vi "configure channel.vi"(7 "EthernetIP configuration":refnum<class "EIP Tags Configuration.lvclass">, 8 "error in":errorcluster, 10 "line item in":T2, 11 "engine configuration in":refnum<class "engine configuration.lvclass">) -> (0 "error out":errorcluster, 1 "success":bool, 2 "line item out":T2, 5 "changed":bool)   [LabVIEW 2013, in "EIP Tags editor node.lvclass"]
uses:
  EIP Tags editor node.lvclass
  table line.ctl
  channel/EIP Tags Channel.lvclass
  <vilib>/NI/Module Execution Interface/Engine Configuration/engine configuration.lvclass
  configuration/EIP Tags Configuration.lvclass
  tag direction.ctl
  configuration/EIP Tags Configuration.lvclass/EIP Tags Configuration.ctl
  <vilib>/NI/Configuration Framework/serializable configuration/NISE_CEF_serializable configuration.lvclass/NISE_CEF_serializable configuration.ctl
  <vilib>/NI/Tag Bus Module Framework/channel/channel classification.ctl
  <vilib>/NI/Tag Bus Module Framework/channel/TBM channel.lvclass/TBM channel.ctl
  <vilib>/NI/Tag Bus/tag/tag descriptor.lvclass/tag descriptor.ctl
  channel/EIP Tags Channel.lvclass/EIP Tags Channel.ctl
  <vilib>/NI/Tag Bus/tag/Data Type.ctl
  configuration/Read EIP tags.vi
  <vilib>/NI/Configuration Framework/serializable configuration/Read UID.vi
  <vilib>/NI/Tag Bus Module Framework/channel/Read channel classification.vi
  <vilib>/NI/Tag Bus/tag/read tag name.vi
  channel/Read element.vi
  channel/Read EIP Tag UUID.vi
  <vilib>/NI/Tag Bus/tag/write tag name.vi
  <vilib>/NI/Tag Bus Module Framework/channel/Write channel classification.vi
  channel/Write EIP Tag UUID.vi
  <vilib>/NI/Tag Bus/tag/read data type.vi
  <vilib>/NI/Tag Bus/tag/write data type.vi
  channel/Write element.vi
  <vilib>/Utility/LVClass/Get LV Class Name.vi
  <vilib>/NI/Configuration Framework/error generator.vi
  <vilib>/NI/Tag Bus Module Framework/channel/TBM channel.lvclass
  <vilib>/NI/Tag Bus/tag/tag descriptor.lvclass
panel:
  in  "Store full array":bool
  in  "direction":T1
  in  "refresh tags":bool
  in  "TBDF Tag":i32(listbox)
  in  "EIP Tag":i32(listbox)
  out "problem":string
  in  "Element Index":i32
  in  "Channel Name":string
  in  "cancel":bool
  in  "ok":bool
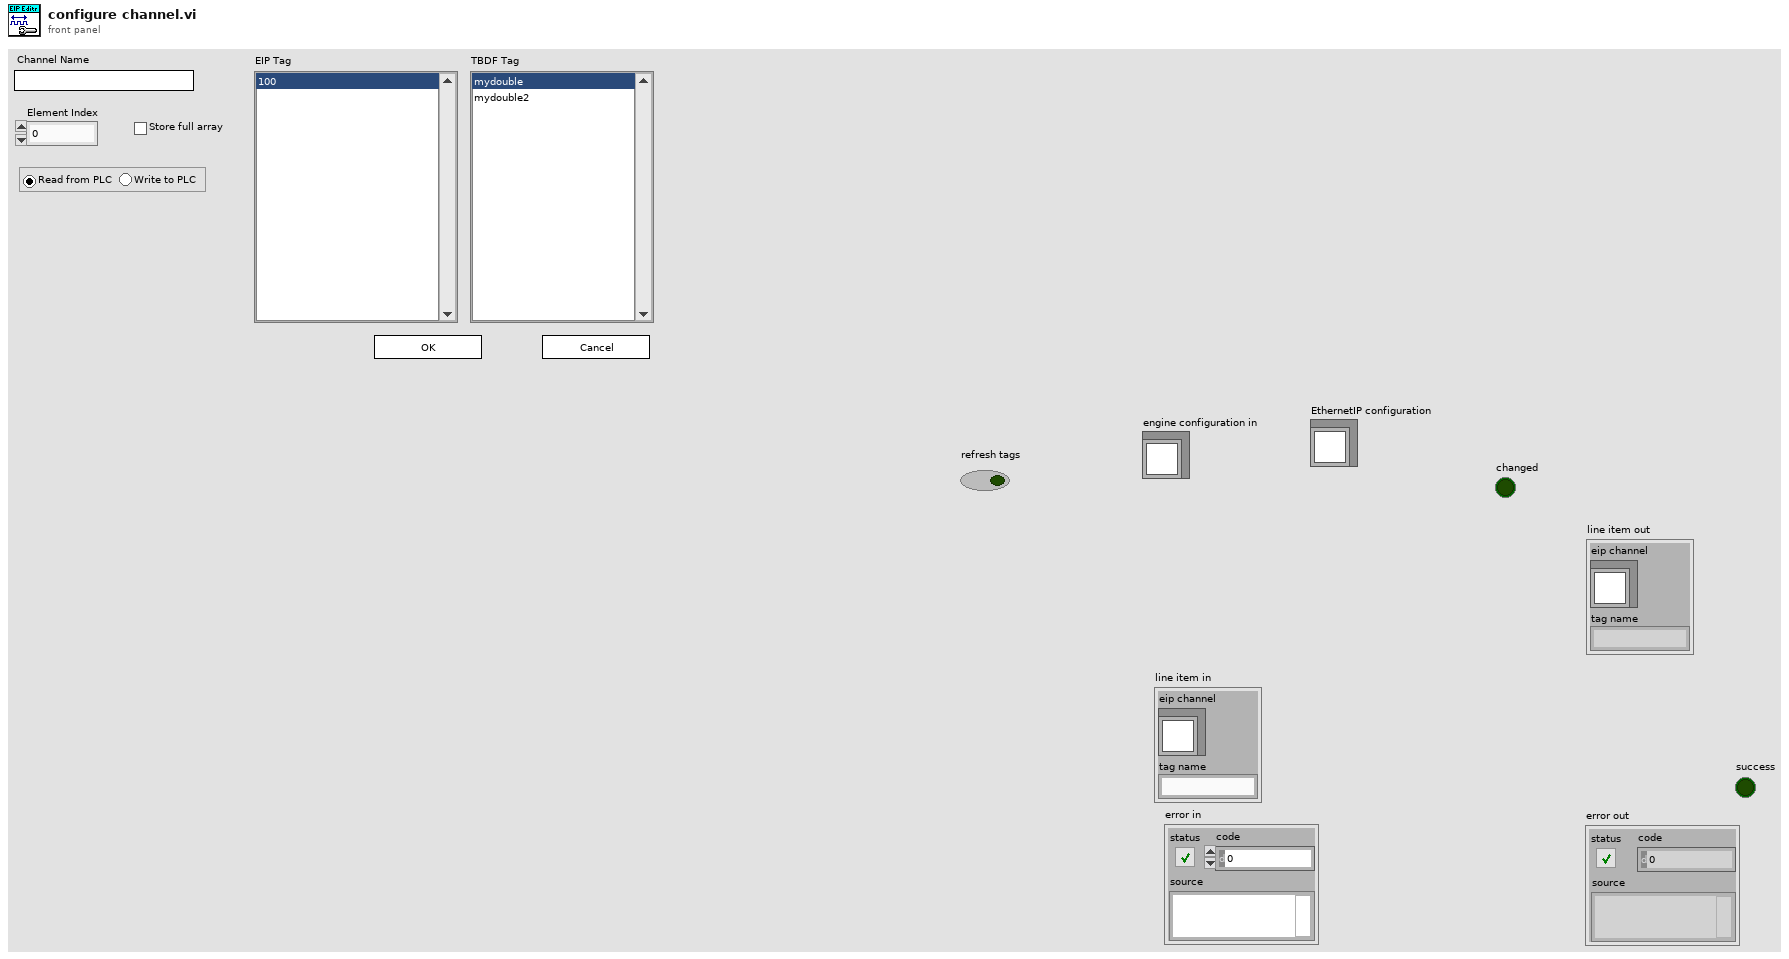
[diagram p1: front panel]
types:
  T1 = typedef "EIP Tags editor node.lvclass/tag direction.ctl" = enum32{"Read from PLC", "Write to PLC"}
  T2 = typedef "EIP Tags editor node.lvclass/table line.ctl" = cluster{"eip channel":refnum<class "EIP Tags Channel.lvclass">, "tag name":string}
  T3 = enum32{"Invalid", "Standard", "Closed", "Hidden", "Minimized", "Maximized"}
  T4 = enum32{"Invalid", "Default", "Floating", "Floating/Auto-Hide", "Modal"}
  T5 = typedef "TBM channel.lvclass/channel classification.ctl" = enum16{"input data", "output data", "processing parameter", "processing result"}
  T6 = enum8{"Enabled", "Disabled", "Disabled and Grayed Out"}
  T7 = typedef "tag bus.lvlib/tag descriptor.lvclass/Data Type.ctl" = enum16{"Double", "Single", "I64", "I32", "I16", "I8", "U64", "U32", "U16", "U8", "Boolean", "String", "Array of Double", "Array of Single", "Array of I64", "Array of I32", "Array of I16", "Array of I8", "Array of U64", "Array of U32", "Array of U16", "Array of U8", "Array of Boolean", "Array of String"}
  T8 = typedef "EIP Tags Configuration.lvclass/eip tag definition.ctl" = cluster{"eip tag types":T9, "unique tag name":string, "Number of Elements":u32}
  T9 = typedef "EIP Tags Configuration.lvclass/eip tag types.ctl" = enum16{"SINT", "INT", "DINT", "REAL", "BOOL", "STRING"}
  T10 = cluster{"unique tag name":string, "tag spec":T8}[]
  T11 = enum32{"invalid app kind", "Development System", "Run Time System", "Student Edition", "Embedded LabVIEW", "Evaluation", "Custom"}
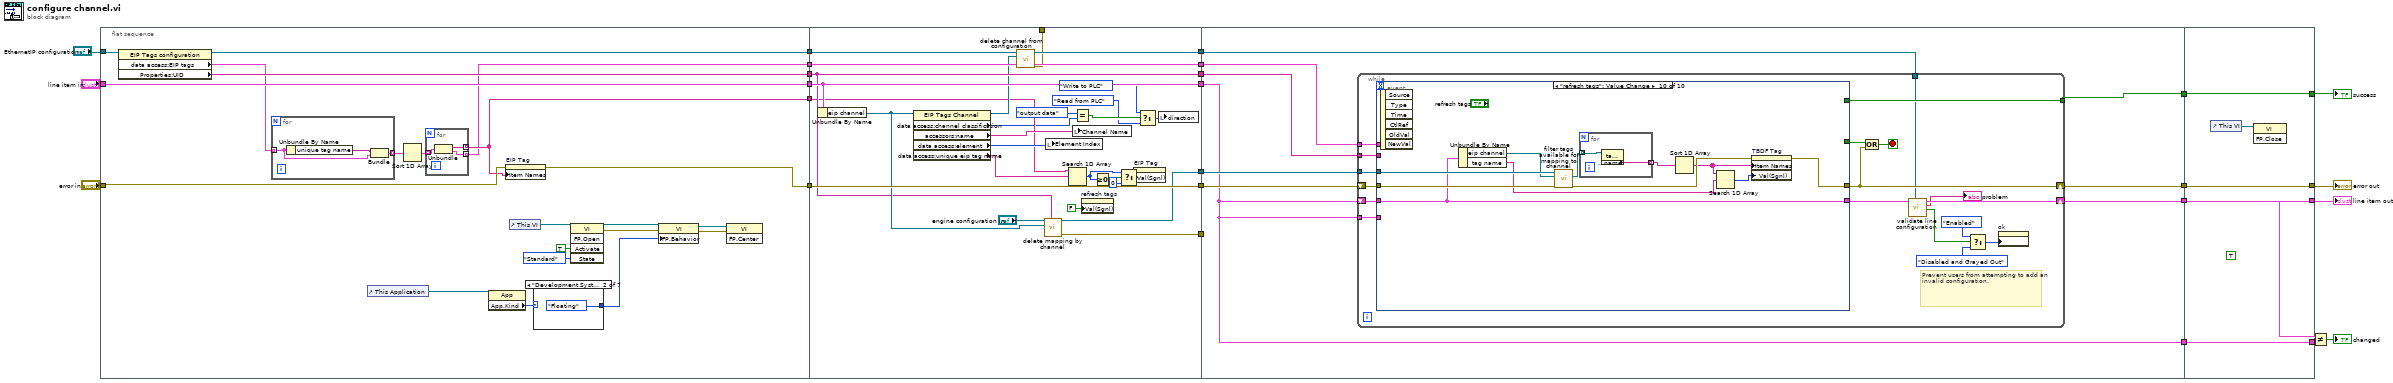
[diagram p0: block diagram]
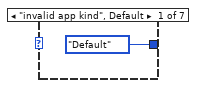
[diagram p2: hidden frame]
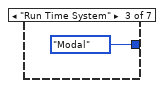
[diagram p3: hidden frame]
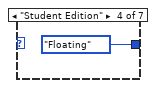
[diagram p4: hidden frame]
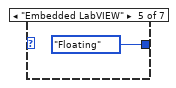
[diagram p5: hidden frame]
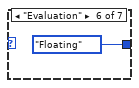
[diagram p6: hidden frame]
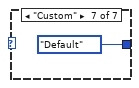
[diagram p7: hidden frame]
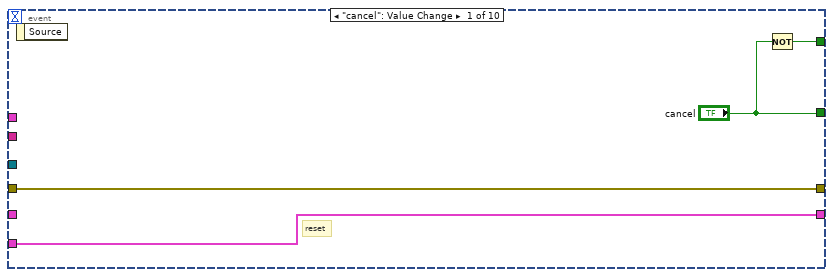
[diagram p8: hidden frame]
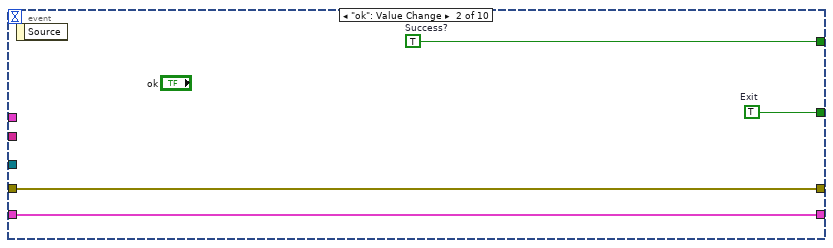
[diagram p9: hidden frame]
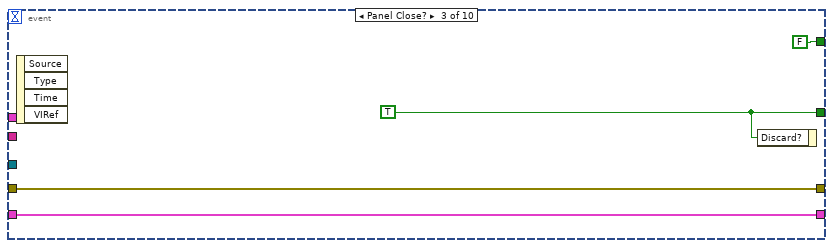
[diagram p10: hidden frame]
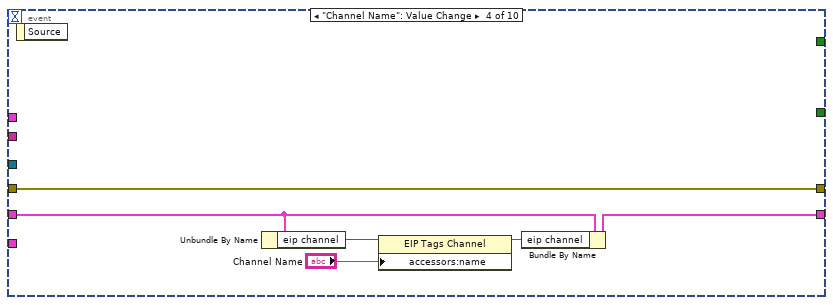
[diagram p11: hidden frame]
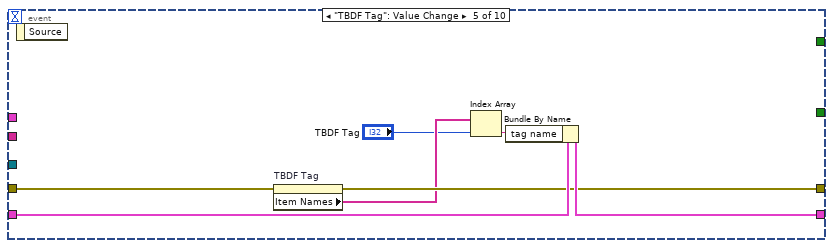
[diagram p12: hidden frame]
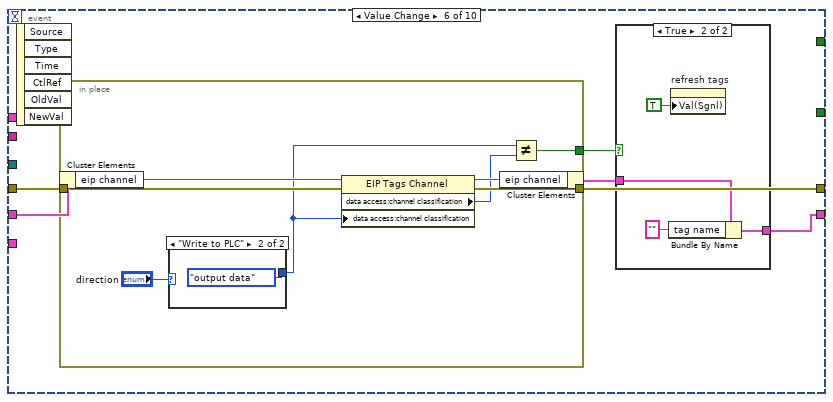
[diagram p13: hidden frame]
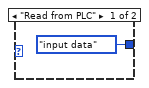
[diagram p15: hidden frame]
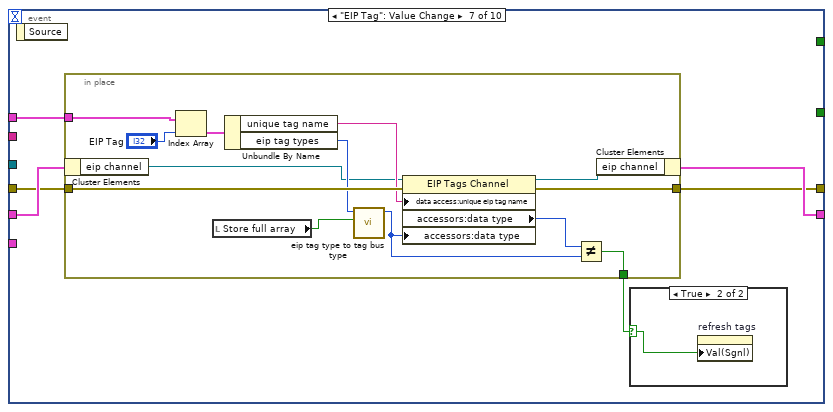
[diagram p16: hidden frame]
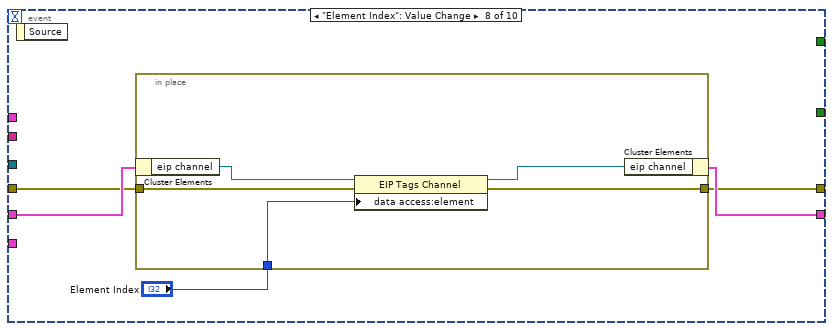
[diagram p18: hidden frame]
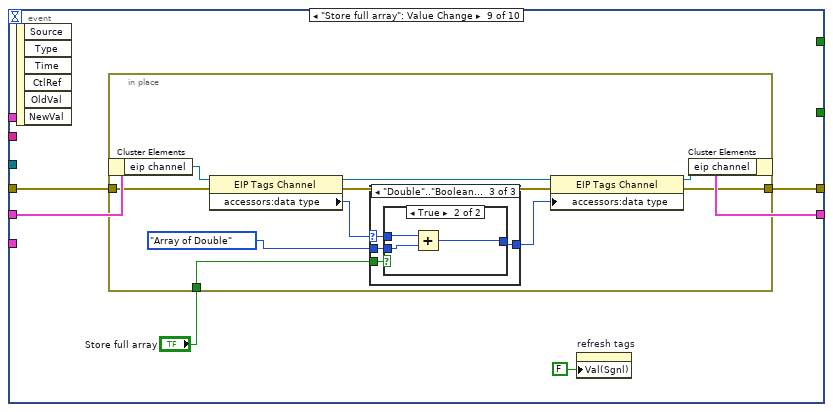
[diagram p19: hidden frame]
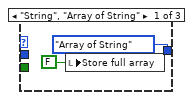
[diagram p20: hidden frame]
diagram:
  n1 = flat-sequence {
    tunnel: "line item in" -> [w46]
    tunnel: "error in" -> [w34]
    tunnel: [w33] -> w14
    tunnel: [w46] -> w12
    tunnel: "EthernetIP configuration" -> [w37]
    tunnel: [w36] -> w6
    tunnel: [w26] -> w4
    tunnel: [w35] -> w3
    tunnel: [w28] -> w1
    tunnel: w14 -> [w86]
    tunnel: [w86] -> w13
    tunnel: w12 -> [w84]
    tunnel: [w84] -> w11
    tunnel: [w82] -> w10
    tunnel: [w81] -> w9
    tunnel: [w75] -> w7
    tunnel: w6 -> [w78]
    tunnel: [w77] -> w5
    tunnel: w4 -> [w77]
    tunnel: w3 -> [w76]
    tunnel: [w76] -> w2
    tunnel: [w73] -> _
    tunnel: w1 -> [w67]
    tunnel: [w94] -> w18
    tunnel: [w93] -> w17
    tunnel: [w92] -> w16
    tunnel: [w87] -> w15
    tunnel: w13 -> [w95]
    tunnel: w11 -> [w87]
    tunnel: w10 -> [_]
    tunnel: w9 -> [w91]
    tunnel: w7 -> [w90]
    tunnel: w5 -> [w89]
    tunnel: w2 -> [w88]
    tunnel: [w237] -> w19
    tunnel: [w238] -> w22
    tunnel: [w239] -> w23
    tunnel: [w240] -> w24
    tunnel: w18 -> [w240]
    tunnel: w17 -> [w239]
    tunnel: w16 -> [w238]
    tunnel: w15 -> [w237]
    frame #0 {
      n2 = property class="EIP Tags configuration"(reference=w37) -> (reference out=w36:refnum<class "EIP Tags Configuration.lvclass">, "data access:EIP tags"=w27:T8[], "Properties:UID"=w35:string)  [unwired: 1 in, 1 out]
      n3 = for {
        tunnel: w27 -> [w51] mode=indexing
        tunnel: [w50] -> w30 mode=indexing
        n4 = Unbundle By Name(w51) -> ("unique tag name"=w52:string)
        n5 = Bundle("unique tag name"=w52, "tag spec"=w51) -> (w50:cluster{"unique tag name":string, "tag spec":T8})  [unwired: 1 in]
      }
      n6 = control-ref of="This Application"() -> (w40:refnum<vi>)
      n7 = Sort 1D Array(array=w30) -> (sorted array=w29:T10)
      n8 = for {
        tunnel: w29 -> [w49] mode=indexing
        tunnel: [w48] -> w28 mode=indexing
        tunnel: [w47] -> w26 mode=indexing
        n9 = Unbundle(w49) -> ("unique tag name"=w48:string, "tag spec"=w47:T8)
      }
      n10 = property class="App"(reference=w40) -> ("App.Kind"=w39:T11)  [unwired: 1 in, 2 out]
      n11 = property on="EIP Tag" class="LstBox (strict)"(error in=w34, "Item Names"=w28) -> (error out=w33:errorcluster)  [unwired: 1 in, 1 out]
      n12 = control-ref of="This VI"() -> (w41:refnum<vi>)
      n13 = case shown="\"Development System\"" w39 {
        tunnel: [T4."Default" ("Front Panel Window:Behavior") T4."Floating" ("Front Panel Window:Behavior") T4."Modal" ("Front Panel Window:Behavior") T4."Floating" ("Front Panel Window:Behavior") T4."Floating" ("Front Panel Window:Behavior") T4."Floating" ("Front Panel Window:Behavior") T4."Default" ("Front Panel Window:Behavior")] -> w38
        frame "invalid app kind", Default {
        }
        frame "Development System" {
        }
        frame "Run Time System" {
        }
        frame "Student Edition" {
        }
        frame "Embedded LabVIEW" {
        }
        frame "Evaluation" {
        }
        frame "Custom" {
        }
      }
      n14 = invoke class="VI" method="FP.Open"(reference=w41, "Activate"=TRUE ("Activate?"), "State"=T3."Standard") -> (reference out=w44:refnum<vi>, error out=w45:errorcluster)  [unwired: 2 in, 3 out]
      n15 = property class="VI"(reference=w44, error in=w45, "FP.Behavior"=w38) -> (reference out=w32:refnum<vi>, error out=w31:errorcluster)
      n16 = invoke class="VI" method="FP.Center"(reference=w32, error in=w31) -> ()  [unwired: 1 in, 3 out]
    }
    frame #1 {
      n17 = Unbundle By Name(w84) -> ("eip channel"=w80:refnum<class "EIP Tags Channel.lvclass">)
      n18 = property class="EIP Tags Channel"(reference=w80) -> (reference out=w74:refnum<class "EIP Tags Channel.lvclass">, "data access:channel classification"=w65:T5, "accessors:name"=w85:string, "data access:element"=w79:i32, "data access:unique eip tag name"=w66:string)  [unwired: 1 in, 1 out]
      n19 = call "delete channel from configuration.vi"("TBM channel in"=w74, "EthernetIP configuration in"=w78) -> ("error out"=w73:errorcluster, "EthernetIP configuration out"=w75:refnum<class "EIP Tags Configuration.lvclass">)  [unwired: 8 in]
      n20 = call <vilib>:"delete mapping by channel.vi"("owner ID"=w76, "channel"=w80, "engine configuration in"="engine configuration in") -> ("error out"=w82:errorcluster, "engine configuration out"=w81:refnum<class "engine configuration.lvclass">)  [unwired: 7 in]
      n21 = local write "Element Index"(w79) -> ()
      n22 = Search 1D Array(1D array=w67, element=w66) -> (index of element=w70:i32)  [unwired: 1 in]
      n23 = local write "Channel Name"(w85) -> ()
      n24 = Equal?(x=channel_classification."output data", y=w65) -> (x = y?=w63:bool)
      n25 = property on="refresh tags" class="Bool (strict)"("Val(Sgnl)"=FALSE ("Value (Signaling)")) -> ()  [unwired: 2 in, 2 out]
      n26 = Greater Or Equal To 0?(x=w70) -> (x >= 0?=w71:bool)
      n27 = Select(t=w70, s=w71, f=0) -> (s? t:f=w69:i32)
      n28 = property on="EIP Tag" class="LstBox (strict)"("Val(Sgnl)"=w69) -> ()  [unwired: 2 in, 2 out]
      n29 = Select(t=tag_direction."Write to PLC" ("direction"), s=w63, f=tag_direction."Read from PLC" ("direction")) -> (s? t:f=w62:T1)
      n30 = local write "direction"(w62) -> ()
    }
    frame #2 {
      n31 = while {
        shift-right: [w104] -> w93
        shift-left: w95 -> [w112]
        tunnel: [w111] -> w94
        shift-right: [w105] -> w92
        shift-left: w87 -> [w108]
        tunnel: w87 -> [w107]
        tunnel: w91 -> [w113]
        tunnel: w90 -> [w99]
        tunnel: w89 -> [w98]
        tunnel: w88 -> [w97]
        stop <- w109 stop-if-true
        # "Prevent users from attempting to add an invalid configuration."
        n32 = event shown="[9] \"refresh tags\": Value Change" {
          selector: _ -> [_ _ _ _ _ _ _ _ _ _]
          dyn-events: _ -> [_ _ _ _ _ _ _ _ _ _]
          timeout: _ -> [_ _ _ _ _ _ _ _ _ _]
          tunnel: w113 -> [_ _ _ _ _ _ _ _ _ w231]
          tunnel: w112 -> [w117 w121 w125 w131 w137 w143 w163 w182 w193 w233]
          tunnel: [w117 w121 w125 w131 w134 w142 w162 w181 w192 w232] -> w104
          tunnel: [w116 w118 FALSE _ _ _ _ _ _ _] -> w111
          tunnel: ["cancel" w119 w123 _ _ _ _ _ _ _] -> w110
          tunnel: w108 -> [_ w120 w122 w129 w138 w144 w165 w184 w195 w230]
          tunnel: [w114 w120 w122 w130 w136 w139 w164 w183 w194 w230] -> w106
          tunnel: w107 -> [w114 _ _ _ _ _ _ _ _ _]
          tunnel: w98 -> [_ _ _ _ _ _ w160 _ _ _]
          tunnel: w97 -> [_ _ _ _ _ _ _ _ _ _]
          event "cancel": Value Change {
            # "reset"
            n33 = event-data() -> ()  [unwired: 1 in, 1 out]
            n34 = Not(x="cancel") -> (.not. x?=w116:bool)
          }
          event "ok": Value Change {
            w118 = TRUE  # Success?
            w119 = TRUE  # Exit
            n35 = event-data() -> ()  [unwired: 1 in, 1 out]
          }
          event Panel Close? {
            w123 = TRUE ("cancel")
            n36 = event-data() -> ()  [unwired: 1 in, 4 out]
            n37 = event-data("Discard?"=w123) -> ()  [unwired: 1 in, 1 out]
          }
          event "Channel Name": Value Change {
            n38 = event-data() -> ()  [unwired: 1 in, 1 out]
            n39 = Unbundle By Name(w129) -> ("eip channel"=w128:refnum<class "EIP Tags Channel.lvclass">)
            n40 = property class="EIP Tags Channel"(reference=w128, "accessors:name"="Channel Name") -> (reference out=w127:refnum<class "EIP Tags Channel.lvclass">)  [unwired: 1 in, 1 out]
            n41 = Bundle By Name(cluster=w129, "eip channel"=w127) -> (w130:T2)
          }
          event "TBDF Tag": Value Change {
            n42 = event-data() -> ()  [unwired: 1 in, 1 out]
            n43 = property on="TBDF Tag" class="LstBox (strict)"(error in=w137) -> (error out=w134:errorcluster, "Item Names"=w133:string[])  [unwired: 1 in, 1 out]
            n44 = Index Array(array=w133, index="TBDF Tag") -> (element=w135:string)
            n45 = Bundle By Name(cluster=w138, "tag name"=w135) -> (w136:T2)
          }
          event Value Change {
            n46 = event-data() -> ()  [unwired: 1 in, 6 out]
            n47 = in-place {
              in-place-border: w143 -> [w156]
              in-place-border: [w155] -> w142
              in-place-border: [w152] -> w141
              n48 = in-place-cluster #1(w144) -> ("eip channel"=w157:refnum<class "EIP Tags Channel.lvclass">)
              n49 = case shown="\"Write to PLC\"" "direction" {
                tunnel: [channel_classification."input data" ("channel classification") channel_classification."output data" ("channel classification")] -> w150
                frame "Read from PLC" {
                }
                frame "Write to PLC" {
                }
              }
              n50 = property class="EIP Tags Channel"(reference=w157, error in=w156, "data access:channel classification"=w150) -> (reference out=w154:refnum<class "EIP Tags Channel.lvclass">, error out=w155:errorcluster, "data access:channel classification"=w153:T5)
              n51 = in-place-cluster #1("eip channel"=w154) -> (w140:T2)
              n52 = Not Equal?(x=w150, y=w153) -> (x != y?=w152:bool)
            }
            n53 = case shown="True" w141 {
              tunnel: w140 -> [w145 w148]
              tunnel: [w145 w147] -> w139
              frame False {
              }
              frame True {
                n54 = Bundle By Name(cluster=w148, "tag name"="") -> (w147:T2)
                n55 = property on="refresh tags" class="Bool (strict)"("Val(Sgnl)"=TRUE ("Value (Signaling)")) -> ()  [unwired: 2 in, 2 out]
              }
            }
          }
          event "EIP Tag": Value Change {
            n56 = event-data() -> ()  [unwired: 1 in, 1 out]
            n57 = in-place {
              in-place-border: w163 -> [w179]
              in-place-border: [w178] -> w162
              in-place-border: [w175] -> w161
              in-place-border: w160 -> [w173]
              n58 = in-place-cluster #2(w165) -> ("eip channel"=w167:refnum<class "EIP Tags Channel.lvclass">)
              n59 = Index Array(array=w173, index="EIP Tag") -> (element=w172:T8)
              n60 = local read "Store full array"() -> (w168:bool)
              n61 = Unbundle By Name(w172) -> ("unique tag name"=w171:string, "eip tag types"=w170:T9)
              n62 = call "eip tag type to tag bus type.vi"("array?"=w168, "eip tag types"=w170) -> ("data type"=w169:T7)  [unwired: 9 in]
              n63 = property class="EIP Tags Channel"(reference=w167, error in=w179, "data access:unique eip tag name"=w171, "accessors:data type"=w169) -> (reference out=w177:refnum<class "EIP Tags Channel.lvclass">, error out=w178:errorcluster, "accessors:data type"=w176:T7)
              n64 = Not Equal?(x=w176, y=w169) -> (x != y?=w175:bool)
              n65 = in-place-cluster #2("eip channel"=w177) -> (w164:T2)
            }
            n66 = case shown="True" w161 {
              selector: w161 -> [_ w166]
              frame False {
              }
              frame True {
                n67 = property on="refresh tags" class="Bool (strict)"("Val(Sgnl)"=w166) -> ()  [unwired: 2 in, 2 out]
              }
            }
          }
          event "Element Index": Value Change {
            n68 = event-data() -> ()  [unwired: 1 in, 1 out]
            n69 = in-place {
              in-place-border: w182 -> [w189]
              in-place-border: [w188] -> w181
              in-place-border: "Element Index" -> [w185]
              n70 = in-place-cluster #3(w184) -> ("eip channel"=w187:refnum<class "EIP Tags Channel.lvclass">)
              n71 = property class="EIP Tags Channel"(reference=w187, error in=w189, "data access:element"=w185) -> (reference out=w186:refnum<class "EIP Tags Channel.lvclass">, error out=w188:errorcluster)
              n72 = in-place-cluster #3("eip channel"=w186) -> (w183:T2)
            }
          }
          event "Store full array": Value Change {
            n73 = event-data() -> ()  [unwired: 1 in, 6 out]
            n74 = in-place {
              in-place-border: w193 -> [w205]
              in-place-border: [w202] -> w192
              in-place-border: "Store full array" -> [w197]
              n75 = in-place-cluster #4(w195) -> ("eip channel"=w203:refnum<class "EIP Tags Channel.lvclass">)
              n76 = property class="EIP Tags Channel"(reference=w203, error in=w205) -> (reference out=w201:refnum<class "EIP Tags Channel.lvclass">, error out=w204:errorcluster, "accessors:data type"=w199:T7)
              n77 = case shown="\"Double\"..\"Boolean\"" w199 {
                selector: w199 -> [_ w209 w217]
                tunnel: [Data_Type."Array of String" ("accessors:data type") w210 w218] -> w198
                tunnel: w197 -> [_ w211 w219]
                tunnel: Data_Type."Array of Double" ("data type") -> [_ w208 w216]
                frame "String", "Array of String" {
                  n78 = local write "Store full array"(FALSE ("Store full array")) -> ()
                }
                frame "Array of Double".."Array of Boolean" {
                  n79 = case shown="False" w211 {
                    tunnel: [w212 w215] -> w210
                    tunnel: w209 -> [w214 w215]
                    tunnel: w208 -> [w213 _]
                    frame False {
                      n80 = Subtract(x=w214, y=w213) -> (x-y=w212:u16)
                    }
                    frame True {
                    }
                  }
                }
                frame "Double".."Boolean" {
                  n81 = case shown="True" w219 {
                    tunnel: [w220 w221] -> w218
                    tunnel: w217 -> [w220 w223]
                    tunnel: w216 -> [_ w222]
                    frame False {
                    }
                    frame True {
                      n82 = Add(x=w223, y=w222) -> (x+y=w221:u16)
                    }
                  }
                }
              }
              n83 = property class="EIP Tags Channel"(reference=w201, error in=w204, "accessors:data type"=w198) -> (reference out=w200:refnum<class "EIP Tags Channel.lvclass">, error out=w202:errorcluster)
              n84 = in-place-cluster #4("eip channel"=w200) -> (w194:T2)
            }
            n85 = property on="refresh tags" class="Bool (strict)"("Val(Sgnl)"=FALSE ("Value (Signaling)")) -> ()  [unwired: 2 in, 2 out]
          }
          event "refresh tags": Value Change {
            n86 = event-data() -> ()  [unwired: 1 in, 6 out]
            n87 = Unbundle By Name(w230) -> ("eip channel"=w229:refnum<class "EIP Tags Channel.lvclass">, "tag name"=w226:string)
            n88 = call <vilib>:"filter tags available for mapping to channel.vi"("channel to map to"=w229, "engine configuration in"=w231) -> ("filtered tags"=w228:refnum<class "tag descriptor.lvclass">[])  [unwired: 8 in, 1 out]
            n89 = for {
              tunnel: w228 -> [w235] mode=indexing
              tunnel: [w234] -> w227 mode=indexing
              n90 = property class="tag descriptor"(reference=w235) -> ("accessors:name"=w234:string)  [unwired: 1 in, 2 out]
            }
            n91 = Sort 1D Array(array=w227) -> (sorted array=w224:string[])
            n92 = Search 1D Array(1D array=w224, element=w226) -> (index of element=w225:i32)  [unwired: 1 in]
            n93 = property on="TBDF Tag" class="LstBox (strict)"(error in=w233, "Item Names"=w224, "Val(Sgnl)"=w225) -> (error out=w232:errorcluster)  [unwired: 1 in, 1 out]
          }
        }
        n94 = Compound Arithmetic op=OR(w110, w104) -> (w109:bool)
        n95 = call "validate line configuration.vi"("EthernetIP configuration"=w99, "line in"=w106) -> ("valid?"=w103:bool, "problem"=→"problem":string, "line out"=w105:T2)  [unwired: 7 in]
        n96 = Select(t=T6."Enabled" ("Disabled"), s=w103, f=T6."Disabled and Grayed Out") -> (s? t:f=w100:T6)
        n97 = property on="ok" class="Bool"("DisabledEnum"=w100) -> ()  [unwired: 2 in, 2 out]
      }
    }
    frame #3 {
      (unwired) TRUE ("Visible")
      n98 = control-ref of="This VI"() -> (w236:refnum<vi>)
      n99 = invoke class="VI" method="FP.Close"(reference=w236) -> ()  [unwired: 2 in, 3 out]
    }
  }
  n100 = Not Equal?(x=w22, y=w19) -> (x != y?=→"changed":bool)
  "error out" <- w23
  "success" <- w24
  "line item out" <- w22
